vi "act_4-conv_C_F.vi"() -> ()   [LabVIEW 2010]
panel:
  out "deg F":dbl
  in  "deg C":dbl
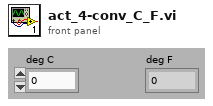
[diagram p1: front panel]
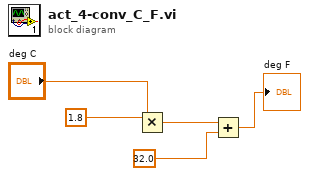
[diagram p0: block diagram]
diagram:
  n1 = Multiply(x=1.8, y="deg C") -> (x*y=w1:dbl)
  n2 = Add(x=w1, y=32.0) -> (x+y=→"deg F":dbl)
